vi "Periodic Tasks.vi"(8 "error in":errorcluster) -> ()   [LabVIEW 2020]
doc: "This VI runs in parallel to other tasks. It can contain as many user-defined periodic loops as you need. These can carry out PID or other sorts of timed response."
uses:
  Trajectory Utilities/DRIVE_PID_TUNING.ctl
  Controls/RobotStates.ctl
  Controls/AimingStates.ctl
  <vilib>/Rock Robotics/WPI/DriverStation/WPI_DriverStationRobotMode2.ctl
  <vilib>/Rock Robotics/WPI/ThirdParty/Phoenix-LabVIEW/Motor Controller/Controls/CTRE_Phoenix_MotorControl_ControlMode.ctl
  <vilib>/Rock Robotics/WPI/ThirdParty/REV Robotics/REVLib/Typedef/Spark MAX Control Type.ctl
  <vilib>/Rock Robotics/WPI/Solenoid/WPI_SolenoidValue.ctl
  Robot Global Data.vi
  Global Variable/Trajectory Variables.vi
  Global Variable/Axes_N_Buttons.vi
  Global Variable/Actuators_N_Sensors.vi
  <vilib>/Rock Robotics/Network Tables/NT Read Number.vi
  Global Variable/LimelightVariables.vi
  <vilib>/Rock Robotics/Network Tables/NT Write Number.vi
  <vilib>/Rock Robotics/WPI/Solenoid/WPI_SolenoidSetEnum.vi
  Global Variable/TurretVariable.vi
  Users/Under Control/Desktop/TrajExamples/FRC_LV_TrajLib_Util_and_Samp-master/Secret_Control_Library_Protected/Secret_Control_Library_Protected.lvlib
  <vilib>/Analysis/NI_AALPro.lvlib
panel:
  in  "Tab Control":T1(tab)=enum."Hood"
  in  "Sensitivty":dbl=1.1
  out "Waveform Chart Turret":T2(graph)
  in  "Gains Turret":enum32{"Limelight Gains", "Encoder Gains"}(tab)
  in  "Turret Gains":T3={"proportional gain (Kc)"=1.0, "integral time (Ti, min)"=0.01, "derivative time (Td, min)"=0.0} {"derivative time (Td, min)" format="%.3f"; "integral time (Ti, min)" format="%.3f"; "proportional gain (Kc)" format="%.3f"}
  in  "Turret Range":cluster{"output high":dbl, "output low":dbl}={"output high"=0.6, "output low"=-0.6} {"output low" format="%.2f"; "output high" format="%.2f"}
  in  "TAIntegral Range":dbl=10000.0
  in  "TADisable Range":dbl
  in  "Deadband LL":dbl
  in  "TADisable Range 2":dbl
  in  "TAIntegral Range 2":dbl=10000.0
  in  "Turret Range 2":cluster{"output high":dbl, "output low":dbl}={"output high"=0.6, "output low"=-0.6} {"output low" format="%.2f"; "output high" format="%.2f"}
  in  "Turret Gains 2":T3={"proportional gain (Kc)"=1.0, "integral time (Ti, min)"=0.01, "derivative time (Td, min)"=0.0} {"derivative time (Td, min)" format="%.3f"; "integral time (Ti, min)" format="%.3f"; "proportional gain (Kc)" format="%.3f"}
  in  "Deadband Encoder":dbl
  out "Turret Output":dbl format="%.2f"
  in  "Enable Aiming":bool
  in  "Setpoint Hood":dbl
  in  "Front Panel Values":bool
  out "Hood Output":dbl format="%.2f"
  out "Waveform Chart Hood":T2(graph)
  in  "Gains Hood":enum32{"Limelight Gains", "Encoder Gains"}(tab)
  in  "Deadband LL 2":dbl
  in  "TADisable Range 4":dbl
  in  "TAIntegral Range 4":dbl=10000.0
  in  "Hood Range":cluster{"output high":dbl, "output low":dbl}={"output high"=0.6, "output low"=-0.6} {"output low" format="%.2f"; "output high" format="%.2f"}
  in  "Hood Gains":T3={"proportional gain (Kc)"=1.0, "integral time (Ti, min)"=0.01, "derivative time (Td, min)"=0.0} {"derivative time (Td, min)" format="%.3f"; "integral time (Ti, min)" format="%.3f"; "proportional gain (Kc)" format="%.3f"}
  in  "Deadband Encoder 2":dbl
  in  "TADisable Range 3":dbl
  in  "TAIntegral Range 3":dbl=10000.0
  in  "Hood Range 2":cluster{"output high":dbl, "output low":dbl}={"output high"=0.6, "output low"=-0.6} {"output low" format="%.2f"; "output high" format="%.2f"}
  in  "Hood Gains 2":T3={"proportional gain (Kc)"=1.0, "integral time (Ti, min)"=0.01, "derivative time (Td, min)"=0.0} {"derivative time (Td, min)" format="%.3f"; "integral time (Ti, min)" format="%.3f"; "proportional gain (Kc)" format="%.3f"}
  in  "Max SP Rate":dbl=30.0
  in  "Max Speed Ft/Sec":dbl=17.0
  in  "Speed PID":T4={"proportional gain  Kp"=0.05, "Integral Gain Ki"=0.0, "Derivative Gain Kd"=0.0}
  out "Left SpeedDmd":dbl
  out "Right SpeedDmd":dbl
  out "TY Limelight":dbl
  in  "Variables":T5
  out "Kicker Value":dbl
  out "Omni Value":dbl
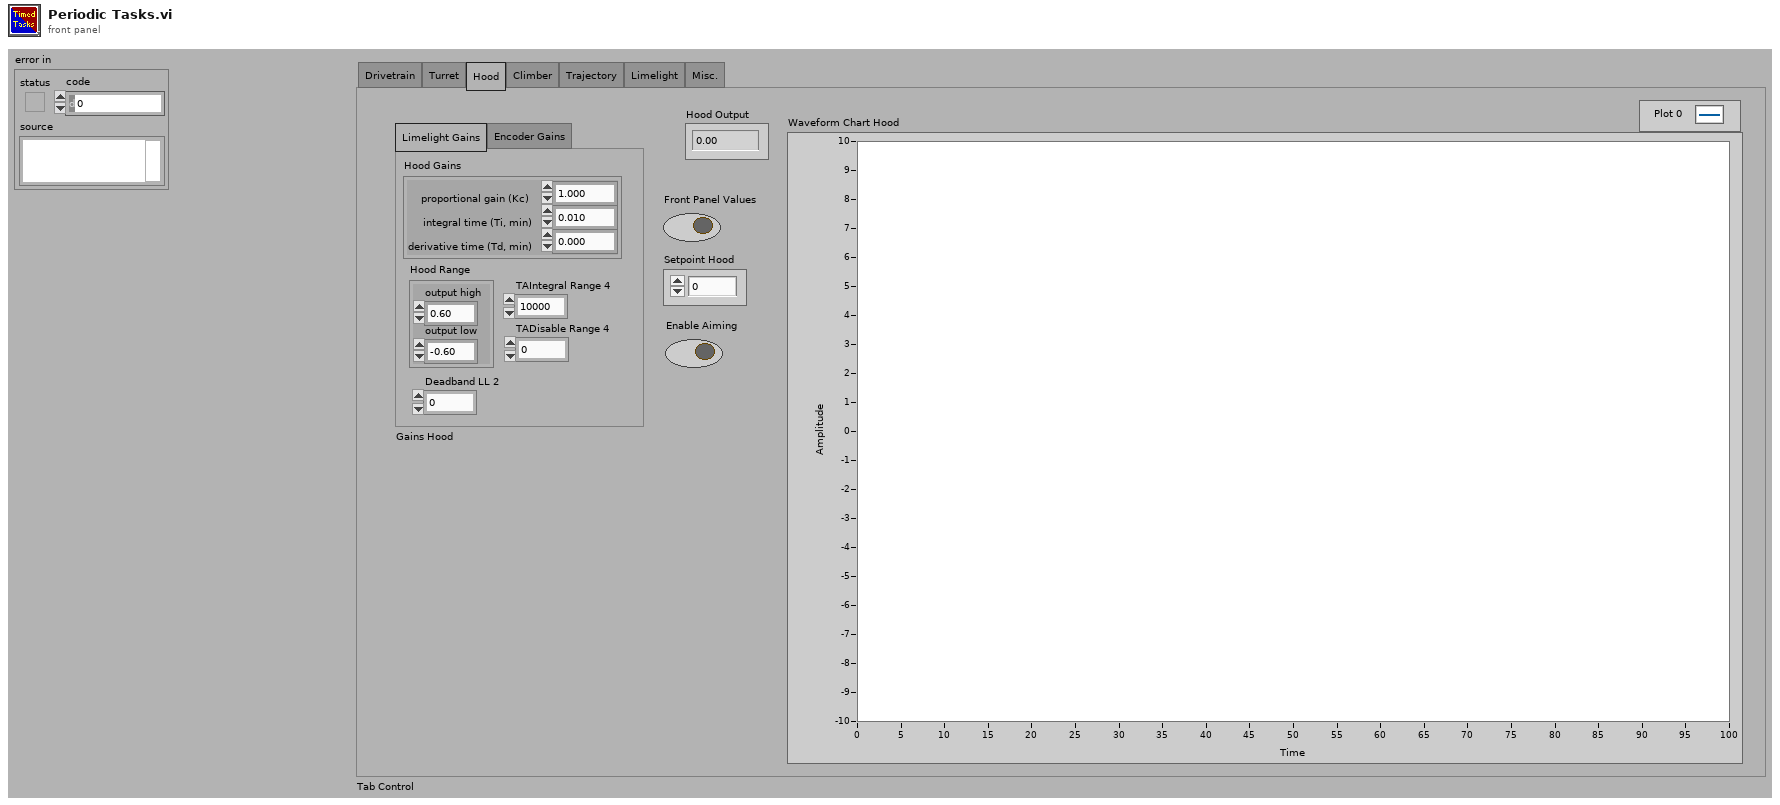
[diagram p1: front panel]
types:
  T1 = enum32{"Drivetrain", "Turret", "Hood", "Climber", "Trajectory", "Limelight", "Misc."}
  T2 = cluster{"EncoderTurretSetpoint":dbl, "offsetAngleX":dbl}
  T3 = cluster{"proportional gain (Kc)":dbl, "integral time (Ti, min)":dbl, "derivative time (Td, min)":dbl}
  T4 = typedef "DRIVE_PID_TUNING.ctl" = cluster{"proportional gain  Kp":dbl, "Integral Gain Ki":dbl, "Derivative Gain Kd":dbl}
  T5 = cluster{"Target Height":dbl, "Mount Angle":dbl, "Len Height":dbl}
  T6 = typedef "AimingStates.ctl" = enum16{"Static", "Aiming to Goal "}
  T7 = typedef "RobotStates.ctl" = enum16{"Default", "Collect Ball", "Prepare Shooting", "Shoot"}
  T8 = typedef "WPI_MotorControlDeviceRef.ctl" = cluster{"DeviceStatus":errorcluster, "Type":T9, "PWM":cluster{"PWM Channel":T10, "DeadBand":T11}, "CAN":cluster{"Device Number":u8, "SetOutput VI Ref":variant, "GetOutput VI Ref":variant, "Enable VI Ref":variant, "Disable VI Ref":variant, "Data":variant}, "Invert":bool, "DIO PWM":cluster{"PWM \"Enable\" Channel":T10, "DIOChannel":T12, "PWM Rate":dbl}}
  T9 = typedef "WPI_MotorControlType.ctl" = enum16{"PWM", "CAN", "DIO PWM"}
  T10 = typedef "FPGA_DIOPWMChannel.ctl" = enum8{"PWM 0", "PWM 1", "PWM 2", "PWM 3", "PWM 4", "PWM 5", "PWM 6", "PWM 7", "PWM 8", "PWM 9", "PWM MXP 0", "PWM MXP 1", "PWM MXP 2", "PWM MXP 3", "PWM MXP 4", "PWM MXP 5", "PWM MXP 6", "PWM MXP 7", "PWM MXP 8", "PWM MXP 9", "Invalid"}
  T11 = typedef "WPI_PWMDeadband.ctl" = cluster{"Name":string, "maxPositivePwm":i32, "minPositivePwm":i32, "centerPwm":i32, "maxNegativePwm":i32, "minNegativePwm":i32, "angularRange":u16}
  T12 = typedef "FPGA_DIOChannel.ctl" = enum8{"DIO 0", "DIO 1", "DIO 2", "DIO 3", "DIO 4", "DIO 5", "DIO 6", "DIO 7", "DIO 8", "DIO 9", "DIO MXP 0", "DIO MXP 1", "DIO MXP 2", "DIO MXP 3", "DIO MXP 4", "DIO MXP 5", "DIO MXP 6", "DIO MXP 7", "DIO MXP 8", "DIO MXP 9", "DIO MXP 10", "DIO MXP 11", "DIO MXP 12", "DIO MXP 13", "DIO MXP 14", "DIO MXP 15", "SPI Port CS1", "SPI Port CS2", "SPI Port CS3", "SPI Port MISO", "SPI Port MOSI", "Invalid"}
  T13 = typedef "WPI_SolenoidDevRef.ctl" = cluster{"DevStatus":errorcluster, "Pneumatics Control Module":u8, "Forward Solenoid Channel":T14, "Reverse Solenoid Channel":T14}
  T14 = typedef "WPI_SolenoidChannel.ctl" = enum8{"Solenoid 0", "Solenoid 1", "Solenoid 2", "Solenoid 3", "Solenoid 4", "Solenoid 5", "Solenoid 6", "Solenoid 7", "Solenoid 8", "Solenoid 9", "Solenoid 10", "Solenoid 11", "Solenoid 12", "Solenoid 13", "Solenoid 14", "Solenoid 15", "Invalid"}
  T15 = typedef "WPI_GyroDevRef.ctl" = cluster{"DevStatus":errorcluster, "Analog Channel":T16, "Gain (VoltsPerDegree/Second)":dbl, "Gyro Type":enum16{"Analog", "XRS450"}, "Handle":i32, "SPI Bus":T17, "Device Found":bool, "Sample Rate":dbl, "Calibrate On Open":bool, "Offset":dbl}
  T16 = typedef "FPGA_AIChannel.ctl" = enum8{"AI 0", "AI 1", "AI 2", "AI 3", "AI MXP 0", "AI MXP 1", "AI MXP 2", "AI MXP 3", "Invalid"}
  T17 = typedef "spi_bus.ctl" = enum16{"SPI On-Board, CS0", "SPI On-Board, CS1", "SPI On-Board, CS2", "SPI On-Board, CS3", "SPI MXP", "Invalid"}
  T18 = typedef "WPI_EncoderDevRef.ctl" = cluster{"DevStatus":errorcluster, "EncoderIndex":T19, "CounterIndex":T20, "DistancePerCount":dbl, "Decoding Type":T21}
  T19 = typedef "FPGA_EncoderIdx.ctl" = enum8{"Enc 0", "Enc 1", "Enc 2", "Enc 3", "Enc 4", "Enc 5", "Enc 6", "Enc 7", "Invalid"}
  T20 = typedef "FPGA_CounterCtrSystemIndex.ctl" = enum8{"Ctr 0", "Ctr 1", "Ctr 2", "Ctr 3", "Ctr 4", "Ctr 5", "Ctr 6", "Ctr 7", "Invalid"}
  T21 = typedef "WPI_EncoderType.ctl" = enum16{"1x", "2x", "4x"}
  T22 = typedef "WPI_SolenoidValue.ctl" = enum16{"Off", "On", "Forward", "Reverse"}
  T23 = typedef "Spark MAX Control Type.ctl" = enum16{"Percent VBus", "Voltage", "Velocity", "Position", "Smart Motion", "Current", "Smart Velocity"}
  T24 = typedef "CTRE_Phoenix_MotorControl_ControlMode.ctl" = u16
  T25 = typedef "WPI_DriverStationRobotMode2.ctl" = enum16{"Autonomous Disabled", "Autonomous Enabled", "Teleop Disabled", "Teleop Enabled", "Disconnected", "Finish", "Test Disabled", "Test Enabled", "Emergency Stopped"}
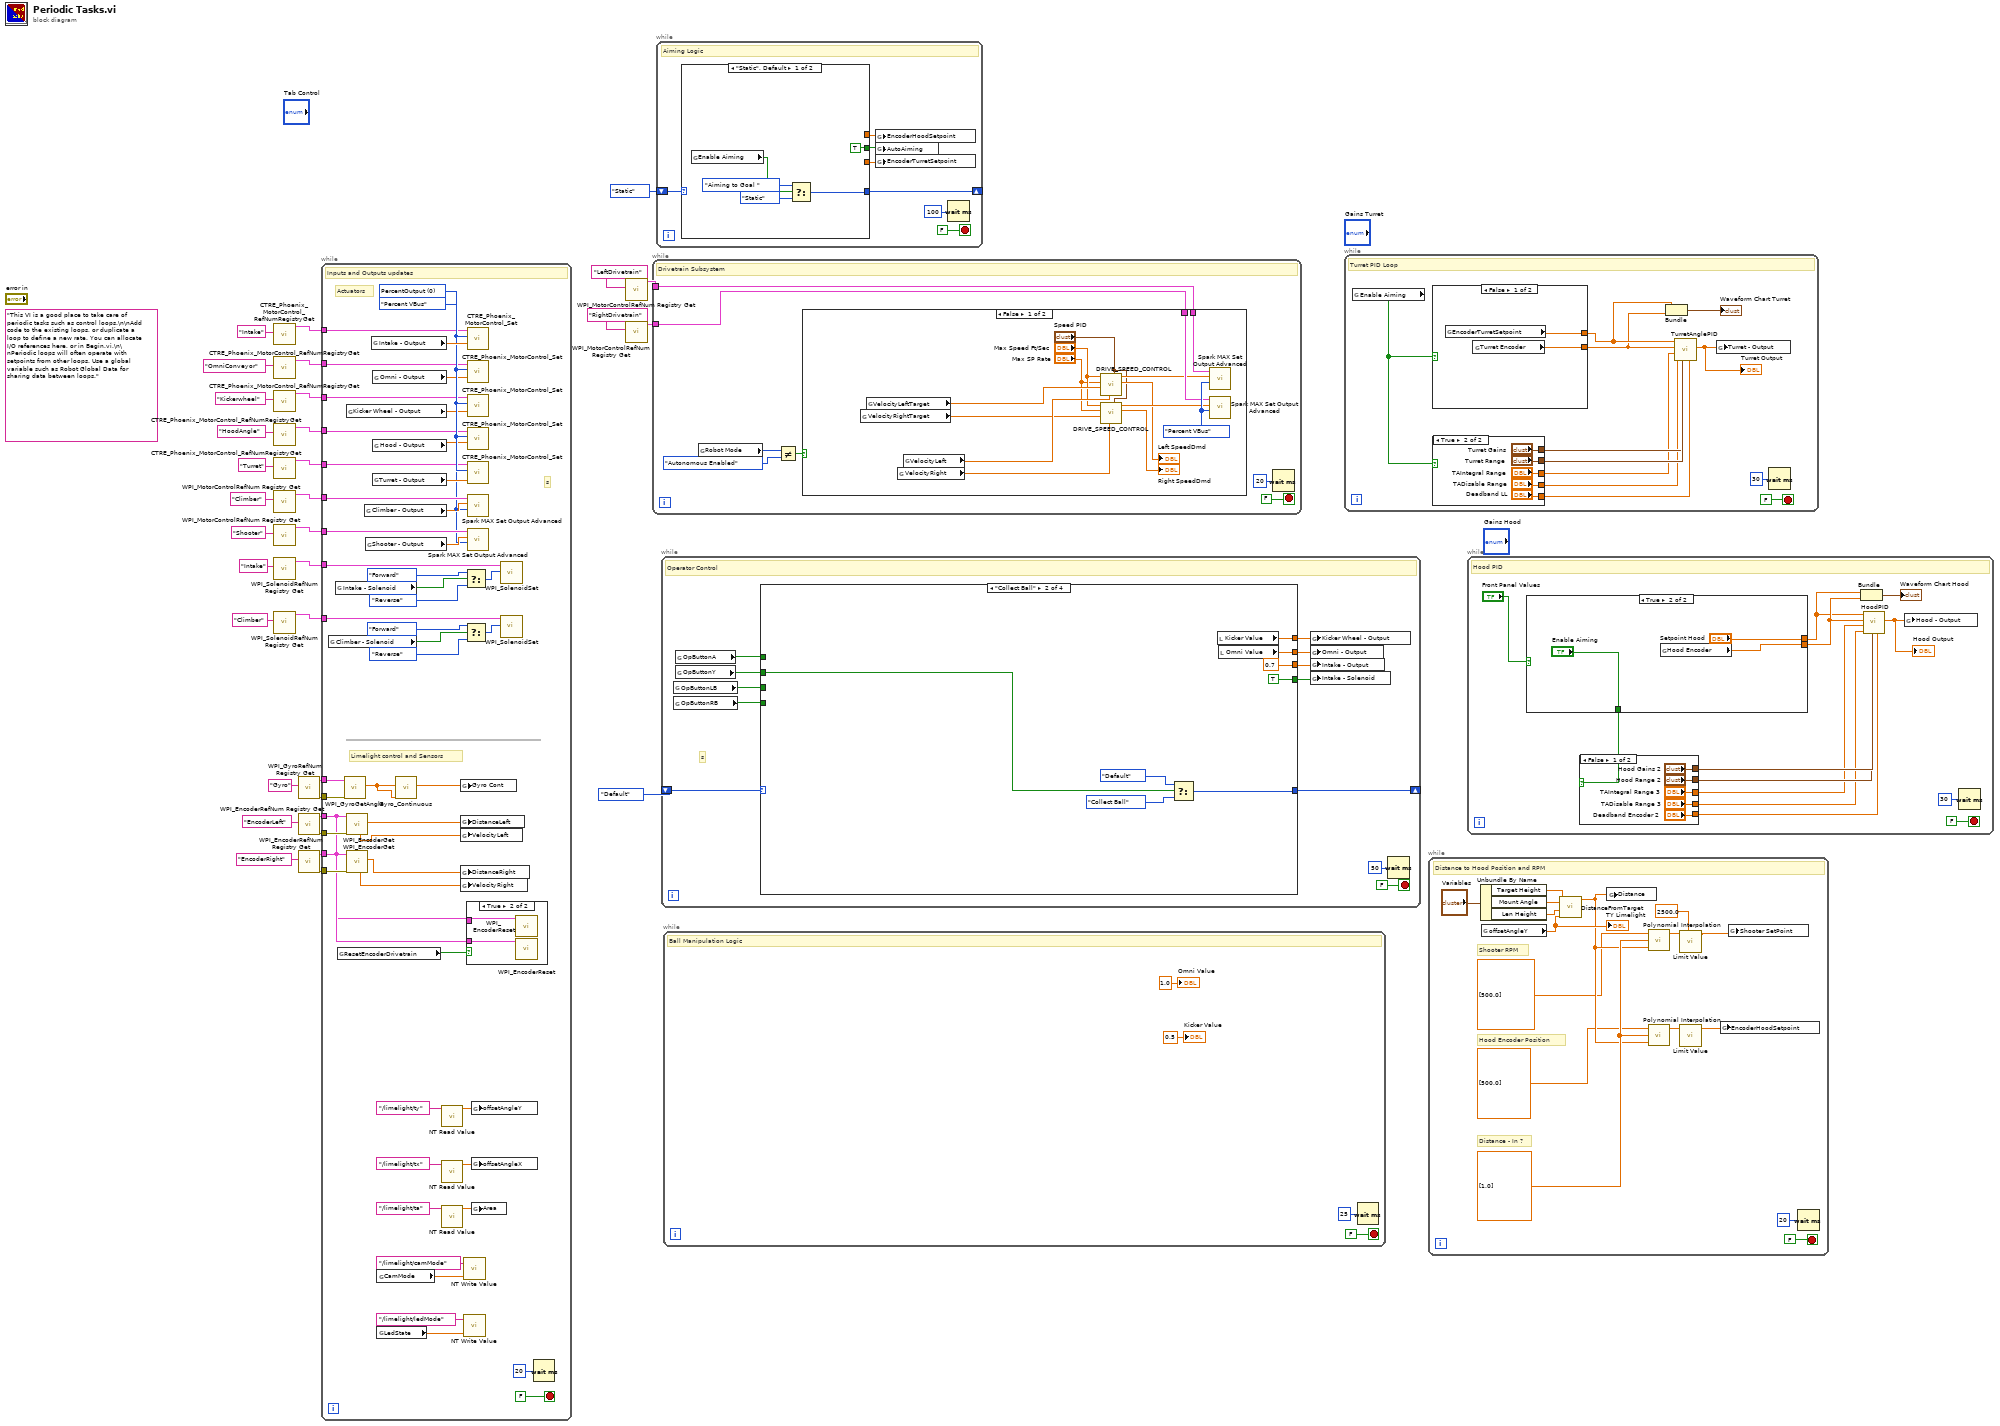
[diagram p0: block diagram]
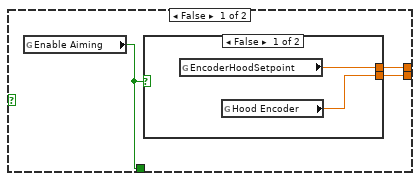
[diagram p2: hidden frame]
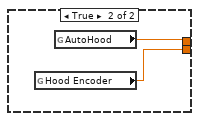
[diagram p3: hidden frame]
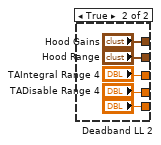
[diagram p4: hidden frame]
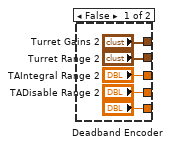
[diagram p5: hidden frame]
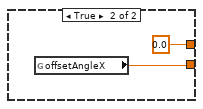
[diagram p6: hidden frame]
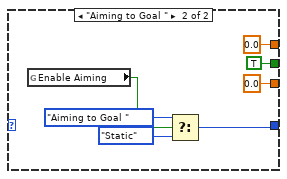
[diagram p7: hidden frame]
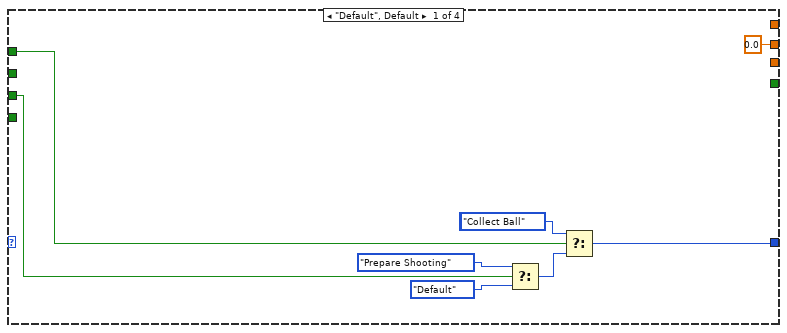
[diagram p8: hidden frame]
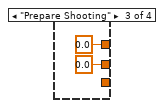
[diagram p9: hidden frame]
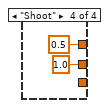
[diagram p10: hidden frame]
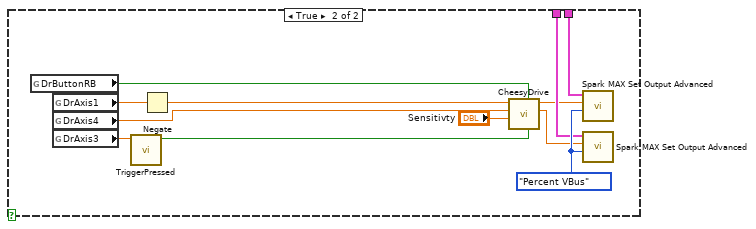
[diagram p11: hidden frame]
diagram:
  (unwired) "This VI is a good place to take care of periodic tasks such as control loops.\n\nAdd code to the existing loops, or duplicate a loop to define a new rate. You can allocate I/O references here, or in Begin.vi.\n\nPeriodic loops will often operate with setpoints from other loops. Use a global variable such as Robot Global Data for sharing data between loops."
  n1 = call <vilib>:"CTRE_Phoenix_MotorControl_RefNumRegistryGet.vi"("refnum name"="Intake") -> ("PhoenixMotorControlDevRef"=w19:T8)  [unwired: 9 in, 1 out]
  n2 = call <vilib>:"CTRE_Phoenix_MotorControl_RefNumRegistryGet.vi"("refnum name"="OmniConveyor") -> ("PhoenixMotorControlDevRef"=w16:T8)  [unwired: 9 in, 1 out]
  n3 = call <vilib>:"CTRE_Phoenix_MotorControl_RefNumRegistryGet.vi"("refnum name"="Kickerwheel") -> ("PhoenixMotorControlDevRef"=w14:T8)  [unwired: 9 in, 1 out]
  n4 = call <vilib>:"CTRE_Phoenix_MotorControl_RefNumRegistryGet.vi"("refnum name"="HoodAngle") -> ("PhoenixMotorControlDevRef"=w12:T8)  [unwired: 9 in, 1 out]
  n5 = call <vilib>:"CTRE_Phoenix_MotorControl_RefNumRegistryGet.vi"("refnum name"="Turret") -> ("PhoenixMotorControlDevRef"=w10:T8)  [unwired: 9 in, 1 out]
  n6 = call <vilib>:"WPI_MotorControlRefNum Registry Get.vi"("refnum name"="Climber") -> ("MotorControlDevRef"=w6:T8)  [unwired: 9 in, 1 out]
  n7 = call <vilib>:"WPI_MotorControlRefNum Registry Get.vi"("refnum name"="Shooter") -> ("MotorControlDevRef"=w7:T8)  [unwired: 9 in, 1 out]
  n8 = call <vilib>:"WPI_SolenoidRefNum Registry Get.vi"("refnum name"="Intake") -> ("SolenoidDevRef"=w3:T13)  [unwired: 9 in, 1 out]
  n9 = call <vilib>:"WPI_SolenoidRefNum Registry Get.vi"("refnum name"="Climber") -> ("SolenoidDevRef"=w2:T13)  [unwired: 9 in, 1 out]
  n10 = call <vilib>:"WPI_GyroRefNum Registry Get.vi"("refnum name"="Gyro") -> ("error out"=w21:errorcluster, "GyroDevRef"=w25:T15)  [unwired: 9 in]
  n11 = call <vilib>:"WPI_EncoderRefNum Registry Get.vi"("refnum name"="EncoderLeft") -> ("error out"=w23:errorcluster, "EncoderDevRef"=w29:T18)  [unwired: 9 in]
  n12 = call <vilib>:"WPI_EncoderRefNum Registry Get.vi"("refnum name"="EncoderRight") -> ("error out"=w22:errorcluster, "EncoderDevRef"=w28:T18)  [unwired: 9 in]
  n13 = while {
    tunnel: w29 -> [w34]
    tunnel: w28 -> [w35]
    tunnel: w25 -> [w72]
    tunnel: w23 -> [w68]
    tunnel: w22 -> [w67]
    tunnel: w21 -> [w66]
    tunnel: w19 -> [w60]
    tunnel: w16 -> [w59]
    tunnel: w14 -> [w56]
    tunnel: w12 -> [w55]
    tunnel: w10 -> [w53]
    tunnel: w7 -> [w51]
    tunnel: w6 -> [w50]
    tunnel: w3 -> [w49]
    tunnel: w2 -> [w48]
    stop <- FALSE stop-if-true
    w45 = Spark_MAX_Control_Type."Percent VBus" ("Control Mode")
    w61 = T24 0 items=["PercentOutput"=0, "Position"=1, "Velocity"=2, "Current"=3, "Follower"=5, "MotionProfile"=6, "MotionMagic"=7, "MotionProfileArc"=10, "Disabled"=15] ("Control Mode")
    # "s"
    # "Actuators"
    # "Limelight control and Sensors"
    # "Inputs and Outputs updates"
    n14 = global read "Actuators_N_Sensors.vi" "Climber - Solenoid"() -> (w40:bool)
    n15 = global read "Actuators_N_Sensors.vi" "Intake - Solenoid"() -> (w44:bool)
    n16 = global read "Actuators_N_Sensors.vi" "ResetEncoderDrivetrain"() -> (w36:bool)
    n17 = call <vilib>:"WPI_GyroGetAngle.vi"("error in (no error)"=w66, "GyroDevRef"=w72) -> ("Angle"=w71:dbl)  [unwired: 5 in, 4 out]
    n18 = global read "Actuators_N_Sensors.vi" "Kicker Wheel - Output"() -> (w57:dbl)
    n19 = call <vilib>:"WPI_EncoderGet.vi"("error in (no error)"=w68, "EncoderDevRef"=w34) -> ("Distance"=w69:dbl, "Rate"=w63:dbl)  [unwired: 4 in, 4 out]
    n20 = call <vilib>:"WPI_EncoderGet.vi"("error in (no error)"=w67, "EncoderDevRef"=w35) -> ("Distance"=w65:dbl, "Rate"=w64:dbl)  [unwired: 4 in, 4 out]
    n21 = global read "Actuators_N_Sensors.vi" "Climber - Output"() -> (w47:dbl)
    n22 = global read "Actuators_N_Sensors.vi" "Shooter - Output"() -> (w46:dbl)
    n23 = global read "Actuators_N_Sensors.vi" "Intake - Output"() -> (w62:dbl)
    n24 = global read "Actuators_N_Sensors.vi" "Turret - Output"() -> (w52:dbl)
    n25 = global read "Actuators_N_Sensors.vi" "Omni - Output"() -> (w58:dbl)
    n26 = global read "Actuators_N_Sensors.vi" "Hood - Output"() -> (w54:dbl)
    n27 = global read "LimelightVariables.vi" "CamMode"() -> (w79:dbl)
    n28 = global read "LimelightVariables.vi" "LedState"() -> (w77:dbl)
    n29 = call "Gyro_Continuous.vi"("GyroInitial"=w71, "GyroInput"=w71) -> ("GyroContinuous"=w70:dbl)  [unwired: 9 in]
    n30 = call-poly <vilib>:"NT Read Value.vi"("Name"="/limelight/ty") -> ("Numeric"=w80:dbl)  [unwired: 9 in, 1 out]
    n31 = call-poly <vilib>:"NT Read Value.vi"("Name"="/limelight/tx") -> ("Numeric"=w82:dbl)  [unwired: 9 in, 1 out]
    n32 = call-poly <vilib>:"NT Read Value.vi"("Name"="/limelight/ta") -> ("Numeric"=w75:dbl)  [unwired: 9 in, 1 out]
    n33 = global write "Trajectory Variables.vi" "Gyro Cont"(w70) -> ()
    n34 = global write "Trajectory Variables.vi" "DistanceLeft"(w69) -> ()
    n35 = global write "Trajectory Variables.vi" "VelocityLeft"(w63) -> ()
    n36 = global write "Trajectory Variables.vi" "DistanceRight"(w65) -> ()
    n37 = global write "Trajectory Variables.vi" "VelocityRight"(w64) -> ()
    n38 = call-poly <vilib>:"NT Write Value.vi"("Numeric"=w79, "Name"="/limelight/camMode") -> ()  [unwired: 9 in, 1 out]
    n39 = call-poly <vilib>:"NT Write Value.vi"("Numeric"=w77, "Name"="/limelight/ledMode") -> ()  [unwired: 9 in, 1 out]
    n40 = Select(t=WPI_SolenoidValue."Forward" ("Value"), s=w44, f=WPI_SolenoidValue."Reverse") -> (s? t:f=w41:T22)
    n41 = Select(t=WPI_SolenoidValue."Forward" ("Value"), s=w40, f=WPI_SolenoidValue."Reverse") -> (s? t:f=w37:T22)
    n42 = case shown="True" w36 {
      tunnel: w35 -> [_ w86]
      tunnel: w34 -> [_ w85]
      frame False {
      }
      frame True {
        n43 = call <vilib>:"WPI_EncoderReset.vi"("EncoderDevRef"=w85) -> ()  [unwired: 9 in, 2 out]
        n44 = call <vilib>:"WPI_EncoderReset.vi"("EncoderDevRef"=w86) -> ()  [unwired: 9 in, 2 out]
      }
    }
    n45 = call <vilib>:"CTRE_Phoenix_MotorControl_Set.vi"("Output"=w62, "Control Mode"=w61, "PhoenixMotorControlDevRef"=w60) -> ()  [unwired: 7 in, 2 out]
    n46 = call <vilib>:"CTRE_Phoenix_MotorControl_Set.vi"("Output"=w58, "Control Mode"=w61, "PhoenixMotorControlDevRef"=w59) -> ()  [unwired: 7 in, 2 out]
    n47 = call <vilib>:"CTRE_Phoenix_MotorControl_Set.vi"("Output"=w57, "Control Mode"=w61, "PhoenixMotorControlDevRef"=w56) -> ()  [unwired: 7 in, 2 out]
    n48 = call <vilib>:"CTRE_Phoenix_MotorControl_Set.vi"("Output"=w54, "Control Mode"=w61, "PhoenixMotorControlDevRef"=w55) -> ()  [unwired: 7 in, 2 out]
    n49 = call <vilib>:"CTRE_Phoenix_MotorControl_Set.vi"("Output"=w52, "Control Mode"=w61, "PhoenixMotorControlDevRef"=w53) -> ()  [unwired: 7 in, 2 out]
    n50 = call <vilib>:"Spark MAX Set Output Advanced.vi"("Control Mode"=w45, "Setpoint"=w47, "MotorControlDevRef"=w50) -> ()  [unwired: 7 in, 2 out]
    n51 = call <vilib>:"Spark MAX Set Output Advanced.vi"("Control Mode"=w45, "Setpoint"=w46, "MotorControlDevRef"=w51) -> ()  [unwired: 7 in, 2 out]
    n52 = global write "LimelightVariables.vi" "offsetAngleY"(w80) -> ()
    n53 = global write "LimelightVariables.vi" "offsetAngleX"(w82) -> ()
    n54 = global write "LimelightVariables.vi" "Area"(w75) -> ()
    n55 = call-poly <vilib>:"WPI_SolenoidSet.vi"("Value"=w41, "SolenoidDevRef"=w49) -> ()  [unwired: 8 in, 2 out]
    n56 = call-poly <vilib>:"WPI_SolenoidSet.vi"("Value"=w37, "SolenoidDevRef"=w48) -> ()  [unwired: 8 in, 2 out]
    n57 = Wait (ms)(milliseconds to wait=u32 20) -> ()  [unwired: 1 out]
  }
  n58 = call <vilib>:"WPI_MotorControlRefNum Registry Get.vi"("refnum name"="LeftDrivetrain") -> ("MotorControlDevRef"=w31:T8)  [unwired: 9 in, 1 out]
  n59 = call <vilib>:"WPI_MotorControlRefNum Registry Get.vi"("refnum name"="RightDrivetrain") -> ("MotorControlDevRef"=w30:T8)  [unwired: 9 in, 1 out]
  n60 = while {
    tunnel: w31 -> [w89]
    tunnel: w30 -> [w88]
    stop <- FALSE stop-if-true
    # "Drivetrain Subsystem"
    n61 = global read "Robot Global Data.vi" "Robot Mode"() -> (w91:T25)
    n62 = Not Equal?(x=w91, y=WPI_DriverStationRobotMode2."Autonomous Enabled") -> (x != y?=w87:bool)
    n63 = case shown="False" w87 {
      tunnel: w89 -> [w106 w117]
      tunnel: w88 -> [w105 w116]
      frame False {
        w107 = Spark_MAX_Control_Type."Percent VBus" ("Control Mode")
        n64 = global read "Trajectory Variables.vi" "VelocityRightTarget"() -> (w102:dbl)
        n65 = global read "Trajectory Variables.vi" "VelocityLeftTarget"() -> (w101:dbl)
        n66 = global read "Trajectory Variables.vi" "VelocityRight"() -> (w104:dbl)
        n67 = global read "Trajectory Variables.vi" "VelocityLeft"() -> (w103:dbl)
        n68 = call "DRIVE_SPEED_CONTROL.vi"("Speed PID"="Speed PID", "Speed (PV)"=w103, "Speed Target (SP)"=w101, "Max SP Rate"="Max SP Rate", "Max Speed Ft/Sec"="Max Speed Ft/Sec") -> ("SpeedDmd"=→"Left SpeedDmd":dbl, "CO-ControlOutput"=w100:dbl)  [unwired: 5 in]
        n69 = call "DRIVE_SPEED_CONTROL.vi"("Speed PID"="Speed PID", "Speed (PV)"=w104, "Speed Target (SP)"=w102, "Max SP Rate"="Max SP Rate", "Max Speed Ft/Sec"="Max Speed Ft/Sec") -> ("SpeedDmd"=→"Right SpeedDmd":dbl, "CO-ControlOutput"=w99:dbl)  [unwired: 5 in]
        n70 = call <vilib>:"Spark MAX Set Output Advanced.vi"("Control Mode"=w107, "Setpoint"=w100, "MotorControlDevRef"=w106) -> ()  [unwired: 7 in, 2 out]
        n71 = call <vilib>:"Spark MAX Set Output Advanced.vi"("Control Mode"=w107, "Setpoint"=w99, "MotorControlDevRef"=w105) -> ()  [unwired: 7 in, 2 out]
      }
      frame True {
        w118 = Spark_MAX_Control_Type."Percent VBus" ("Control Mode")
        n72 = global read "Axes_N_Buttons.vi" "DrButtonRB"() -> (w119:bool)
        n73 = global read "Axes_N_Buttons.vi" "DrAxis1"() -> (w115:dbl)
        n74 = global read "Axes_N_Buttons.vi" "DrAxis4"() -> (w113:dbl)
        n75 = global read "Axes_N_Buttons.vi" "DrAxis3"() -> (w111:dbl)
        n76 = call "TriggerPressed.vi"("Trigger Value"=w111) -> ("Pressed?"=w110:bool)  [unwired: 10 in]
        n77 = Negate(x=w115) -> (-x=w114:dbl)
        n78 = call "CheesyDrive.vi"("SlowRate?"=w110, "Quickturn"=w119, "Sensitivty"="Sensitivty", "Wheel"=w113, "Throttle"=w114) -> ("Right PWM"=w108:dbl, "Left PWM"=w109:dbl)  [unwired: 5 in]
        n79 = call <vilib>:"Spark MAX Set Output Advanced.vi"("Control Mode"=w118, "Setpoint"=w109, "MotorControlDevRef"=w117) -> ()  [unwired: 7 in, 2 out]
        n80 = call <vilib>:"Spark MAX Set Output Advanced.vi"("Control Mode"=w118, "Setpoint"=w108, "MotorControlDevRef"=w116) -> ()  [unwired: 7 in, 2 out]
      }
    }
    n81 = Wait (ms)(milliseconds to wait=u32 20) -> ()  [unwired: 1 out]
  }
  n82 = while {
    shift-right: [w123] -> _
    shift-left: AimingStates."Static" ("Aiming State") -> [w122]
    stop <- FALSE stop-if-true
    # "Aiming Logic"
    n83 = case shown="\"Static\", Default" w122 {
      tunnel: [TRUE ("AutoAiming") TRUE ("AutoAiming")] -> w124
      tunnel: [w127 w133] -> w123
      tunnel: [_ 0.0 ("EncoderTurretSetpoint")] -> w121
      tunnel: [_ 0.0 ("EncoderTurretSetpoint")] -> w120
      frame "Static", Default {
        n84 = global read "TurretVariable.vi" "Enable Aiming"() -> (w130:bool)
        n85 = Select(t=AimingStates."Aiming to Goal " ("Aiming State"), s=w130, f=AimingStates."Static" ("Aiming State")) -> (s? t:f=w127:T6)
      }
      frame "Aiming to Goal " {
        n86 = global read "TurretVariable.vi" "Enable Aiming"() -> (w136:bool)
        n87 = Select(t=AimingStates."Aiming to Goal " ("Aiming State"), s=w136, f=AimingStates."Static" ("Aiming State")) -> (s? t:f=w133:T6)
      }
    }
    n88 = global write "TurretVariable.vi" "EncoderHoodSetpoint"(w120) -> ()
    n89 = global write "TurretVariable.vi" "AutoAiming"(w124) -> ()
    n90 = global write "TurretVariable.vi" "EncoderTurretSetpoint"(w121) -> ()
    n91 = Wait (ms)(milliseconds to wait=u32 100) -> ()  [unwired: 1 out]
  }
  n92 = while {
    shift-right: [w146] -> _
    shift-left: RobotStates."Default" ("Enum") -> [w148]
    stop <- FALSE stop-if-true
    # "s"
    # "Operator Control"
    n93 = global read "Axes_N_Buttons.vi" "OpButtonLB"() -> (w143:bool)
    n94 = global read "Axes_N_Buttons.vi" "OpButtonRB"() -> (w142:bool)
    n95 = global read "Axes_N_Buttons.vi" "OpButtonA"() -> (w147:bool)
    n96 = global read "Axes_N_Buttons.vi" "OpButtonY"() -> (w144:bool)
    n97 = case shown="\"Collect Ball\"" w148 {
      tunnel: w147 -> [w158 _ _ _]
      tunnel: [w156 w162 _ _] -> w146
      tunnel: [_ 0.7 ("Intake - Output") _ _] -> w145
      tunnel: w144 -> [_ w163 _ _]
      tunnel: w143 -> [w155 _ _ _]
      tunnel: w142 -> [_ _ _ _]
      tunnel: [_ TRUE ("Intake - Solenoid") _ _] -> w141
      tunnel: [0.0 ("Quicker Value") w160 0.0 ("Omni Value") 1.0 ("Omni Value")] -> w140
      tunnel: [_ w159 0.0 ("Kicker Value") 0.5 ("Kicker Value")] -> w139
      frame "Default", Default {
        (unwired) RobotStates."Collect Ball" ("Enum")
        n98 = Select(t=RobotStates."Prepare Shooting" ("Enum"), s=w155, f=RobotStates."Default" ("Enum")) -> (s? t:f=w153:T7)
        n99 = Select(t=RobotStates."Collect Ball" ("Enum"), s=w158, f=w153) -> (s? t:f=w156:T7)
      }
      frame "Collect Ball" {
        n100 = Select(t=RobotStates."Default" ("Enum"), s=w163, f=RobotStates."Collect Ball" ("Enum")) -> (s? t:f=w162:T7)
        n101 = local read "Kicker Value"() -> (w159:dbl)
        n102 = local read "Omni Value"() -> (w160:dbl)
      }
      frame "Prepare Shooting" {
      }
      frame "Shoot" {
      }
    }
    n103 = global write "Actuators_N_Sensors.vi" "Kicker Wheel - Output"(w139) -> ()
    n104 = global write "Actuators_N_Sensors.vi" "Omni - Output"(w140) -> ()
    n105 = global write "Actuators_N_Sensors.vi" "Intake - Output"(w145) -> ()
    n106 = global write "Actuators_N_Sensors.vi" "Intake - Solenoid"(w141) -> ()
    n107 = Wait (ms)(milliseconds to wait=u32 50) -> ()  [unwired: 1 out]
  }
  n108 = while {
    stop <- FALSE stop-if-true
    # "Ball Manipulation Logic"
    n109 = Wait (ms)(milliseconds to wait=u32 25) -> ()  [unwired: 1 out]
    "Omni Value" <- 1.0 ("Omni Value")
    "Kicker Value" <- 0.5 ("Kicker Wheel")
  }
  n110 = while {
    stop <- FALSE stop-if-true
    # "Turret PID Loop"
    n111 = global read "TurretVariable.vi" "Enable Aiming"() -> (w182:bool)
    n112 = case shown="False" w182 {
      tunnel: [w197 w200] -> w177
      tunnel: [w198 0.0 ("EncoderTurretSetpoint")] -> w178
      frame False {
        n113 = global read "TurretVariable.vi" "EncoderTurretSetpoint"() -> (w198:dbl)
        n114 = global read "Actuators_N_Sensors.vi" "Turret Encoder"() -> (w197:dbl)
      }
      frame True {
        n115 = global read "LimelightVariables.vi" "offsetAngleX"() -> (w200:dbl)
      }
    }
    n116 = case shown="True" w182 {
      tunnel: ["Turret Range 2" "Turret Range"] -> w184
      tunnel: ["Turret Gains 2" "Turret Gains"] -> w183
      tunnel: ["TADisable Range 2" "TADisable Range"] -> w181
      tunnel: ["TAIntegral Range 2" "TAIntegral Range"] -> w176
      tunnel: ["Deadband Encoder" "Deadband LL"] -> w175
      frame False {
      }
      frame True {
      }
    }
    n117 = Bundle("EncoderTurretSetpoint"=w178, "offsetAngleX"=w177) -> (→"Waveform Chart Turret":T2)  [unwired: 1 in]
    n118 = call "TurretAnglePID.vi"("Deadband"=w175, "TAGains"=w183, "TARange"=w184, "TADisable Range"=w181, "TAIntegral Range"=w176, "TAProcess variable"=w177, "TASetpoint"=w178) -> ("TAoutput"=w180:dbl)  [unwired: 4 in]
    "Turret Output" <- w180
    n119 = global write "Actuators_N_Sensors.vi" "Turret - Output"(w180) -> ()
    n120 = Wait (ms)(milliseconds to wait=u32 30) -> ()  [unwired: 1 out]
  }
  n121 = while {
    stop <- FALSE stop-if-true
    w211 = dbl[] [1.0] ("X")
    # "Shooter RPM"
    # "Hood Encoder Position"
    # "Distance - In ?"
    # "Distance to Hood Position and RPM"
    n122 = Unbundle By Name("Variables") -> ("Target Height"=w214:dbl, "Mount Angle"=w213:dbl, "Len Height"=w212:dbl)
    n123 = global read "LimelightVariables.vi" "offsetAngleY"() -> (w209:dbl)
    "TY Limelight" <- w209
    n124 = call "DistanceFromTarget.vi"("ty Limelight"=w209, "Altura da lente"=w212, "Ângulo de montagem"=w213, "Altura do alvo"=w214) -> ("Distance From the Target"=w208:dbl)  [unwired: 7 in]
    n125 = global write "LimelightVariables.vi" "Distance"(w208) -> ()
    n126 = call <vilib>:"Polynomial Interpolation.vi"("x value"=w208, "X"=w211, "Y"=dbl[] [500.0]) -> ("interpolation value"=w205:dbl)  [unwired: 2 out]
    n127 = call <vilib>:"Polynomial Interpolation.vi"("x value"=w208, "X"=w211, "Y"=dbl[] [500.0]) -> ("interpolation value"=w202:dbl)  [unwired: 2 out]
    n128 = call "Limit Value.vi"("Value"=w205, "Limit"=2500.0) -> ("Limited Value"=w203:dbl)  [unwired: 6 in]
    n129 = call "Limit Value.vi"("Value"=w202) -> ("Limited Value"=w201:dbl)  [unwired: 7 in]
    n130 = global write "TurretVariable.vi" "EncoderHoodSetpoint"(w201) -> ()
    n131 = global write "Actuators_N_Sensors.vi" "Shooter SetPoint"(w203) -> ()
    n132 = Wait (ms)(milliseconds to wait=u32 20) -> ()  [unwired: 1 out]
  }
  n133 = while {
    stop <- FALSE stop-if-true
    # "Hood PID"
    n134 = case shown="True" "Front Panel Values" {
      tunnel: [w232 w239] -> w220
      tunnel: [w231 "Setpoint Hood"] -> w219
      tunnel: [w230 "Enable Aiming"] -> w218
      frame False {
        n135 = global read "TurretVariable.vi" "Enable Aiming"() -> (w230:bool)
        n136 = case shown="False" w230 {
          tunnel: [w234 w235] -> w232
          tunnel: [w233 w236] -> w231
          frame False {
            n137 = global read "TurretVariable.vi" "EncoderHoodSetpoint"() -> (w233:dbl)
            n138 = global read "Actuators_N_Sensors.vi" "Hood Encoder"() -> (w234:dbl)
          }
          frame True {
            n139 = global read "Actuators_N_Sensors.vi" "Hood Encoder"() -> (w235:dbl)
            n140 = global read "TurretVariable.vi" "AutoHood"() -> (w236:dbl)
          }
        }
      }
      frame True {
        n141 = global read "Actuators_N_Sensors.vi" "Hood Encoder"() -> (w239:dbl)
      }
    }
    n142 = case shown="False" w218 {
      tunnel: ["Hood Range 2" "Hood Range"] -> w225
      tunnel: ["Hood Gains 2" "Hood Gains"] -> w226
      tunnel: ["TAIntegral Range 3" "TAIntegral Range 4"] -> w224
      tunnel: ["TADisable Range 3" "TADisable Range 4"] -> w223
      tunnel: ["Deadband Encoder 2" "Deadband LL 2"] -> w222
      frame False {
      }
      frame True {
      }
    }
    n143 = Bundle("Setpoint Hood"=w219, "Hood Encoder"=w220) -> (→"Waveform Chart Hood":cluster{"Setpoint Hood":dbl, "Hood Encoder":dbl})  [unwired: 1 in]
    n144 = call "HoodPID.vi"("Deadband"=w222, "TAGains"=w226, "TARange"=w225, "TADisable Range"=w223, "TAIntegral Range"=w224, "TAProcess variable"=w220, "TASetpoint"=w219) -> ("TAoutput"=w228:dbl)  [unwired: 4 in]
    "Hood Output" <- w228
    n145 = global write "Actuators_N_Sensors.vi" "Hood - Output"(w228) -> ()
    n146 = Wait (ms)(milliseconds to wait=u32 30) -> ()  [unwired: 1 out]
  }
